vi "get run time total.vi"(11 "run Times":T1[](array[typedef])) -> (3 "total time (s)":dbl)   [LabVIEW 2013, in "utf junit report.lvlib"]
uses:
  utf junit report.lvlib
  <vilib>/utf/common/utf_test_result_troll_new.ctl
  <vilib>/utf/common/utf_test_result.ctl
  <vilib>/utf/common/utf_vector_result.ctl
  <vilib>/utf/common/utf_test_result_failure.ctl
  <vilib>/utf/common/utf_test_comparison_operators.ctl
  <vilib>/utf/common/utf_vi_tag.ctl
  <vilib>/utf/common/utf_test_result_input_data.ctl
  <vilib>/utf/NI_UnitTestFramework.lvlib
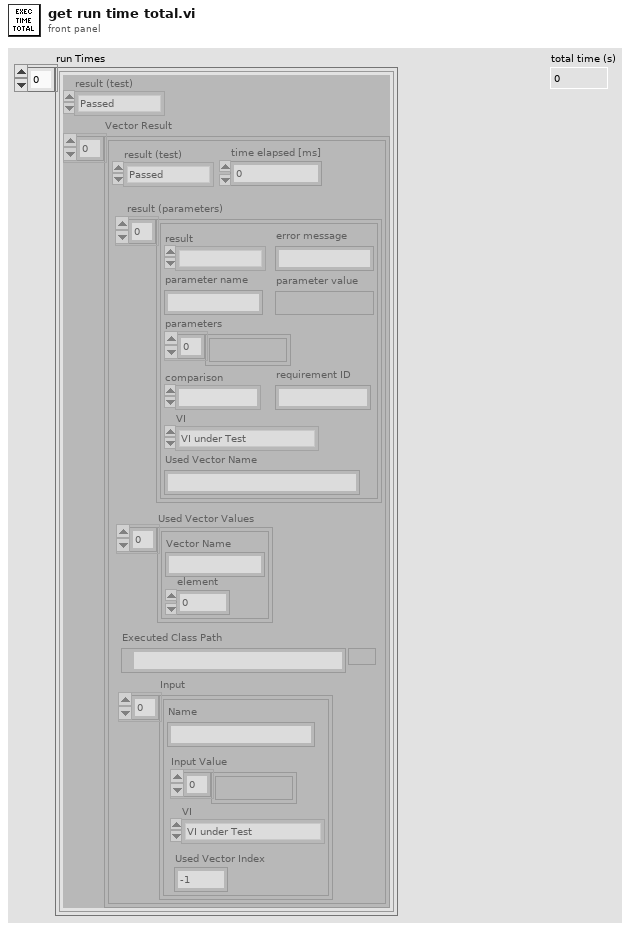
[diagram p1: front panel]
types:
  T1 = typedef "NI_UnitTestFramework.lvlib/utf_test_result_troll_new.ctl" = cluster{"result (test)":T2, "Vector Result":T3[]}
  T2 = typedef "NI_UnitTestFramework.lvlib/utf_test_result.ctl" = enum16{"Passed", "Failed", "Error", "Skipped", "Not Processed"}
  T3 = typedef "NI_UnitTestFramework.lvlib/utf_vector_result.ctl" = cluster{"time elapsed [ms]":u32, "result (test)":T2, "result (parameters)":T4[], "Used Vector Values":cluster{"Vector Name":string, "element":i32}[], "Executed Class Path":path, "Input":T7[]}
  T4 = typedef "NI_UnitTestFramework.lvlib/utf_test_result_failure.ctl" = cluster{"result":T2, "error message":string, "parameter name":string, "parameter value":variant, "parameters":variant[], "comparison":T5, "requirement ID":string, "VI":T6, "Used Vector Name":string}
  T5 = typedef "NI_UnitTestFramework.lvlib/utf_test_comparison_operators.ctl" = enum16{"=", "!=", ">", ">=", "<", "<=", "range", "symmetric tolerance", "asymmetric tolerance", "string contains", "string not contain", "array size", "string length", "array range", "by element", "array range (limit array)", "user-defined", "array contains", "array not contain", "vector length", "= (elm)", "!= (elm)", "= (case insensitive)", "!= (case insensitive)"}
  T6 = typedef "NI_UnitTestFramework.lvlib/utf_vi_tag.ctl" = enum16{"Setup VI", "VI under Test", "Teardown VI"}
  T7 = typedef "NI_UnitTestFramework.lvlib/utf_test_result_input_data.ctl" = cluster{"Name":string, "Input Value":variant[], "VI":T6, "Used Vector Index":i32}
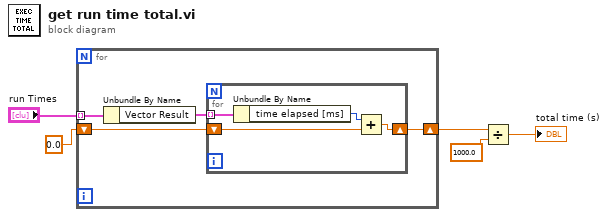
[diagram p0: block diagram]
diagram:
  n1 = for {
    tunnel: "run Times" -> [w9] mode=indexing
    shift-right: [w6] -> w3
    shift-left: 0.0 -> [w7]
    n2 = Unbundle By Name(w9) -> ("Vector Result"=w8:T3[])
    n3 = for {
      tunnel: w8 -> [w13] mode=indexing
      shift-right: [w10] -> w6
      shift-left: w7 -> [w11]
      n4 = Unbundle By Name(w13) -> ("time elapsed [ms]"=w12:u32)
      n5 = Add(x=w12, y=w11) -> (x+y=w10:dbl)
    }
  }
  n6 = Divide(x=w3, y=1000.0) -> (x/y=→"total time (s)":dbl)
